vi "Get Data.vi"(8 "error in":errorcluster, 11 "ePAS in":refnum<class "ePAS.lvclass">) -> (0 "error out":errorcluster, 3 "ePAS out":refnum<class "ePAS.lvclass">)   [LabVIEW 2014, in "ePAS Library.lvlib" / "ePAS.lvclass"]
uses:
  ePAS.lvclass
  reusable/PAS/Data/Main/PAS Data.lvclass
  Data/Cell/ePAS Cell Data.lvclass
  ePAS.lvclass/ePAS.ctl
  reusable/Instrument/Instrument.lvclass/Instrument.ctl
  reusable/PAS/Data/Cell/PAS Cell Data.lvclass/PAS Cell Data.ctl
  Data/Cell/ePAS Cell Data.lvclass/ePAS Cell Data.ctl
  <vilib>/DAQmx/read.llb/DAQmx Read (Analog 2D DBL NChan NSamp).vi
  <vilib>/Analysis/baseanly.llb/Mean (DBL).vi
  reusable/PAS/Data/Cell/Write lRMS.vi
  Data/Cell/Write T.vi
  reusable/Instrument/Read Data.vi
  reusable/Instrument/Write Data.vi
  <vilib>/DAQmx/miscellaneous.llb/DAQmx Fill In Error Info.vi
  <vilib>/Utility/error.llb/Error Cluster From Error Code.vi
  <vilib>/rvi/errors/niLvFpgaAdjustHostInterfaceError.vi
  reusable/PAS/Data/Cell/Write timeData.vi
  reusable/PAS/Data/Cell/Write lasDiodeData.vi
  <vilib>/rvi/interface/nirviMethod/nirviMethod.xnode
  FPGA/R FPGA Ref.ctl
  FPGA Bitfiles/FPGA Server.lvbitx
  reusable/Data/Data.lvclass
  FPGA/Session/Exscalabar FPGA.lvclass
  ePAS Library.lvlib
  reusable/Instrument/Instrument.lvclass
  <vilib>/Analysis/NI_AALBase.lvlib
  <vilib>/FPGAPlugInAG/PXI-7842R/niLvFpga_ReadFifo_PXI-7842R.vi
  <vilib>/rvi/errors/niLvFpgaMergeErrorWithErrorCode.vi
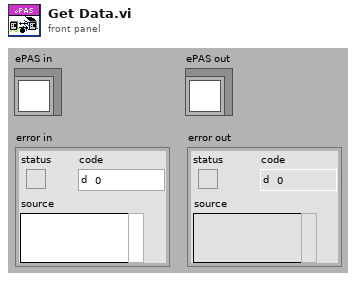
[diagram p1: front panel]
types:
  T1 = typedef "Session - Root.lvclass/Session Handle.ctl" = refnum<data-value>
  T2 = typedef "ePAS Library.lvlib/R FPGA Ref.ctl" = refnum<k20>
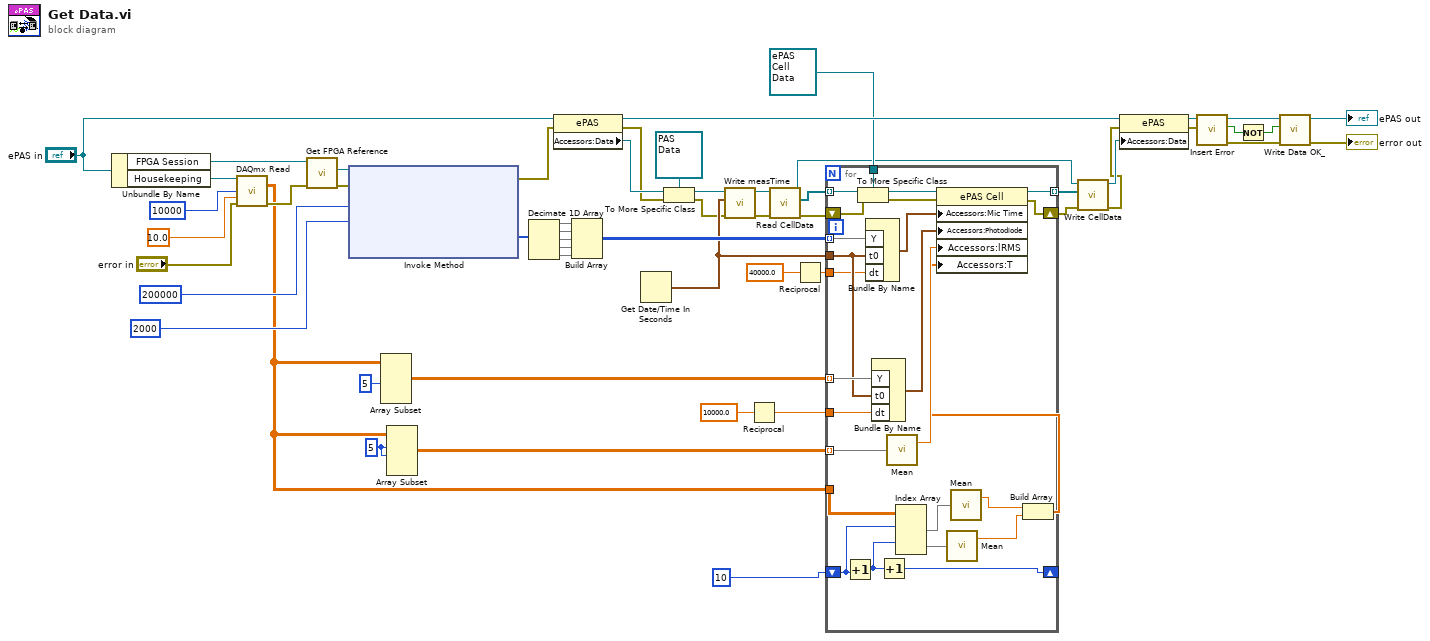
[diagram p0: block diagram]
diagram:
  w13 = 5 ("index")
  n1 = Unbundle By Name("ePAS in") -> ("FPGA Session"=w50:T1, "Housekeeping"=w54:refnum<k21>)
  n2 = call-poly <vilib>:"DAQmx Read.vi"("task/channels in"=w54, "number of samples per channel"=10000, "timeout"=10.0, "error in"="error in") -> ("data"=w2:dbl[][], "error out"=w49:errorcluster)  [unwired: 9 in, 1 out]
  n3 = call "Get FPGA Reference.vi"("error in"=w49, "Session In"=w50) -> ("error out"=w47:errorcluster, "Ex FPGA Ref"=w48:T2)  [unwired: 7 in, 1 out]
  n4 = xnode "Invoke Method"("FPGA VI Reference In"=w48, "error in"=w47, "Number of Elements"=u32 200000, "Timeout (ms)"=2000) -> ("error out"=w18:errorcluster, "Data"=w44:i16[])  [unwired: 2 out]
  n5 = Array Subset(array=w2, length (row)=5 ("length")) -> (w16:dbl[][])  [unwired: 3 in]
  n6 = Array Subset(array=w2, index (row)=w13, length (row)=w13) -> (w12:dbl[][])  [unwired: 2 in]
  n7 = Decimate 1D Array(w44) -> (w43:i16[], w42:i16[], w41:i16[], w40:i16[], w39:i16[])
  n8 = property class="ePAS"(reference="ePAS in", error in=w18) -> (reference out=w22:refnum<class "ePAS.lvclass">, error out=w23:errorcluster, "Accessors:Data"=w26:refnum<class "Data.lvclass">)
  n9 = Build Array(w43, w42, w41, w40, w39) -> (w38:i16[][])
  n10 = Get Date/Time In Seconds() -> (seconds since 1Jan1904=w37:timestamp)
  n11 = To More Specific Class(target class=refnum<class "PAS Data.lvclass"> refnum ("PAS Data"), reference=w26, error in=w23) -> (specific class reference=w24:refnum<class "PAS Data.lvclass">, error out=w19:errorcluster)
  n12 = call "Write measTime.vi"("error in (no error)"=w19, "measTime"=w37, "Data in"=w24) -> ("error out"=w10:errorcluster, "Data out"=w11:refnum<class "PAS Data.lvclass">)  [unwired: 7 in]
  n13 = Reciprocal(x=10000.0) -> (1/x=w14:dbl)
  n14 = call "Read CellData.vi"("error in"=w10, "PAS Data in"=w11) -> ("error out"=w8:errorcluster, "CellData"=w9:refnum<class "PAS Cell Data.lvclass">[], "PAS Data out"=w4:refnum<class "PAS Data.lvclass">)  [unwired: 7 in]
  n15 = Reciprocal(x=40000.0) -> (1/x=w35:dbl)
  n16 = for {
    tunnel: w38 -> [w79] mode=indexing
    tunnel: w37 -> [w76]
    tunnel: w35 -> [w75]
    tunnel: w16 -> [w77] mode=indexing
    tunnel: w14 -> [w74]
    tunnel: w12 -> [w73] mode=indexing
    tunnel: w9 -> [w71] mode=indexing
    tunnel: refnum<class "ePAS Cell Data.lvclass"> refnum ("ePAS Cell Data.lvclass") -> [w67]
    tunnel: [w64] -> w6 mode=indexing
    tunnel: w2 -> [w58]
    shift-right: [w57] -> _
    shift-left: 10 ("index (row)") -> [w56]
    shift-right: [w78] -> w34
    shift-left: w8 -> [w69]
    n17 = Increment(x=w56) -> (x+1=w59:i32)
    n18 = To More Specific Class(target class=w67, reference=w71, error in=w69) -> (specific class reference=w70:refnum<class "ePAS Cell Data.lvclass">, error out=w68:errorcluster)
    n19 = Bundle By Name("Y"=w79, "t0"=w76, "dt"=w75) -> (w72:waveform(i16))  [unwired: 1 in]
    n20 = Bundle By Name("Y"=w77, "t0"=w76, "dt"=w74) -> (w66:waveform(dbl))  [unwired: 1 in]
    n21 = Increment(x=w59) -> (x+1=w57:i32)
    n22 = call-poly <vilib>:"Mean.vi"("X"=w73) -> ("mean"=w65:dbl)  [unwired: 1 out]
    n23 = Index Array(array=w58, index (row) #1=w56, index (row) #2=w59) -> (element #1=w60:dbl[], element #2=w61:dbl[])  [unwired: 2 in]
    n24 = call-poly <vilib>:"Mean.vi"("X"=w61) -> ("mean"=w63:dbl)  [unwired: 1 out]
    n25 = call-poly <vilib>:"Mean.vi"("X"=w60) -> ("mean"=w62:dbl)  [unwired: 1 out]
    n26 = Build Array(w62, w63) -> (w55:dbl[])
    n27 = property class="ePAS Cell"(reference=w70, error in=w68, "Accessors:Mic Time"=w72, "Accessors:Photodiode"=w66, "Accessors:lRMS"=w65, "Accessors:T"=w55) -> (reference out=w64:refnum<class "ePAS Cell Data.lvclass">, error out=w78:errorcluster)
  }
  n28 = call "Write CellData.vi"("error in"=w34, "CellData"=w6, "PAS Data in"=w4) -> ("error out"=w3:errorcluster, "PAS Data out"=w5:refnum<class "PAS Data.lvclass">)  [unwired: 7 in]
  n29 = property class="ePAS"(reference=w22, error in=w3, "Accessors:Data"=w5) -> (reference out=w20:refnum<class "ePAS.lvclass">, error out=w21:errorcluster)
  n30 = call "Insert Error.vi"("err"=w21, "Instrument in"=w20) -> ("error out"=w30:errorcluster, "error?"=w32:bool, "Instrument out"=w33:refnum<class "ePAS.lvclass">)  [unwired: 7 in]
  n31 = Not(x=w32) -> (.not. x?=w31:bool)
  n32 = call "Write Data OK_.vi"("error in (no error)"=w30, "Data OK?"=w31, "Instrument in"=w33) -> ("error out"=→"error out":errorcluster, "Instrument out"=→"ePAS out":refnum<class "ePAS.lvclass">)  [unwired: 7 in]
